vi "RPC Method RouteGuide RecordRoute.vi"(3 "error in (no error)":errorcluster, 4 "gRPCid in":T2, 5 "DNL_LabVIEW Object in":refnum<class "RouteGuideImpl.lvclass">) -> (0 "error out":errorcluster, 1 "gRPCid out":T2, 2 "DNL_LabVIEW Object out":refnum<class "RouteGuideImpl.lvclass">)   [LabVIEW 2019, in "UserCode_impl_server.lvlib" / "RouteGuideImpl.lvclass"]
uses:
  RouteGuideImpl.lvclass
  <vilib>/gRPC/LabVIEW gRPC Library/Shared/grpcId.ctl
  Generated_stub_server/RPC Messages/routeguide_RouteSummary.ctl
  Generated_stub_server/RPC Messages/routeguide_Point.ctl
  Generated_stub_server/Generated_stub_server.lvlib
  Generated_stub_server/RPC Service/RouteGuideStub/RouteGuideStub.lvclass
  <vilib>/gRPC/LabVIEW gRPC Library/grpc-lvsupport-release.lvlib
panel:
  in  "?":T1
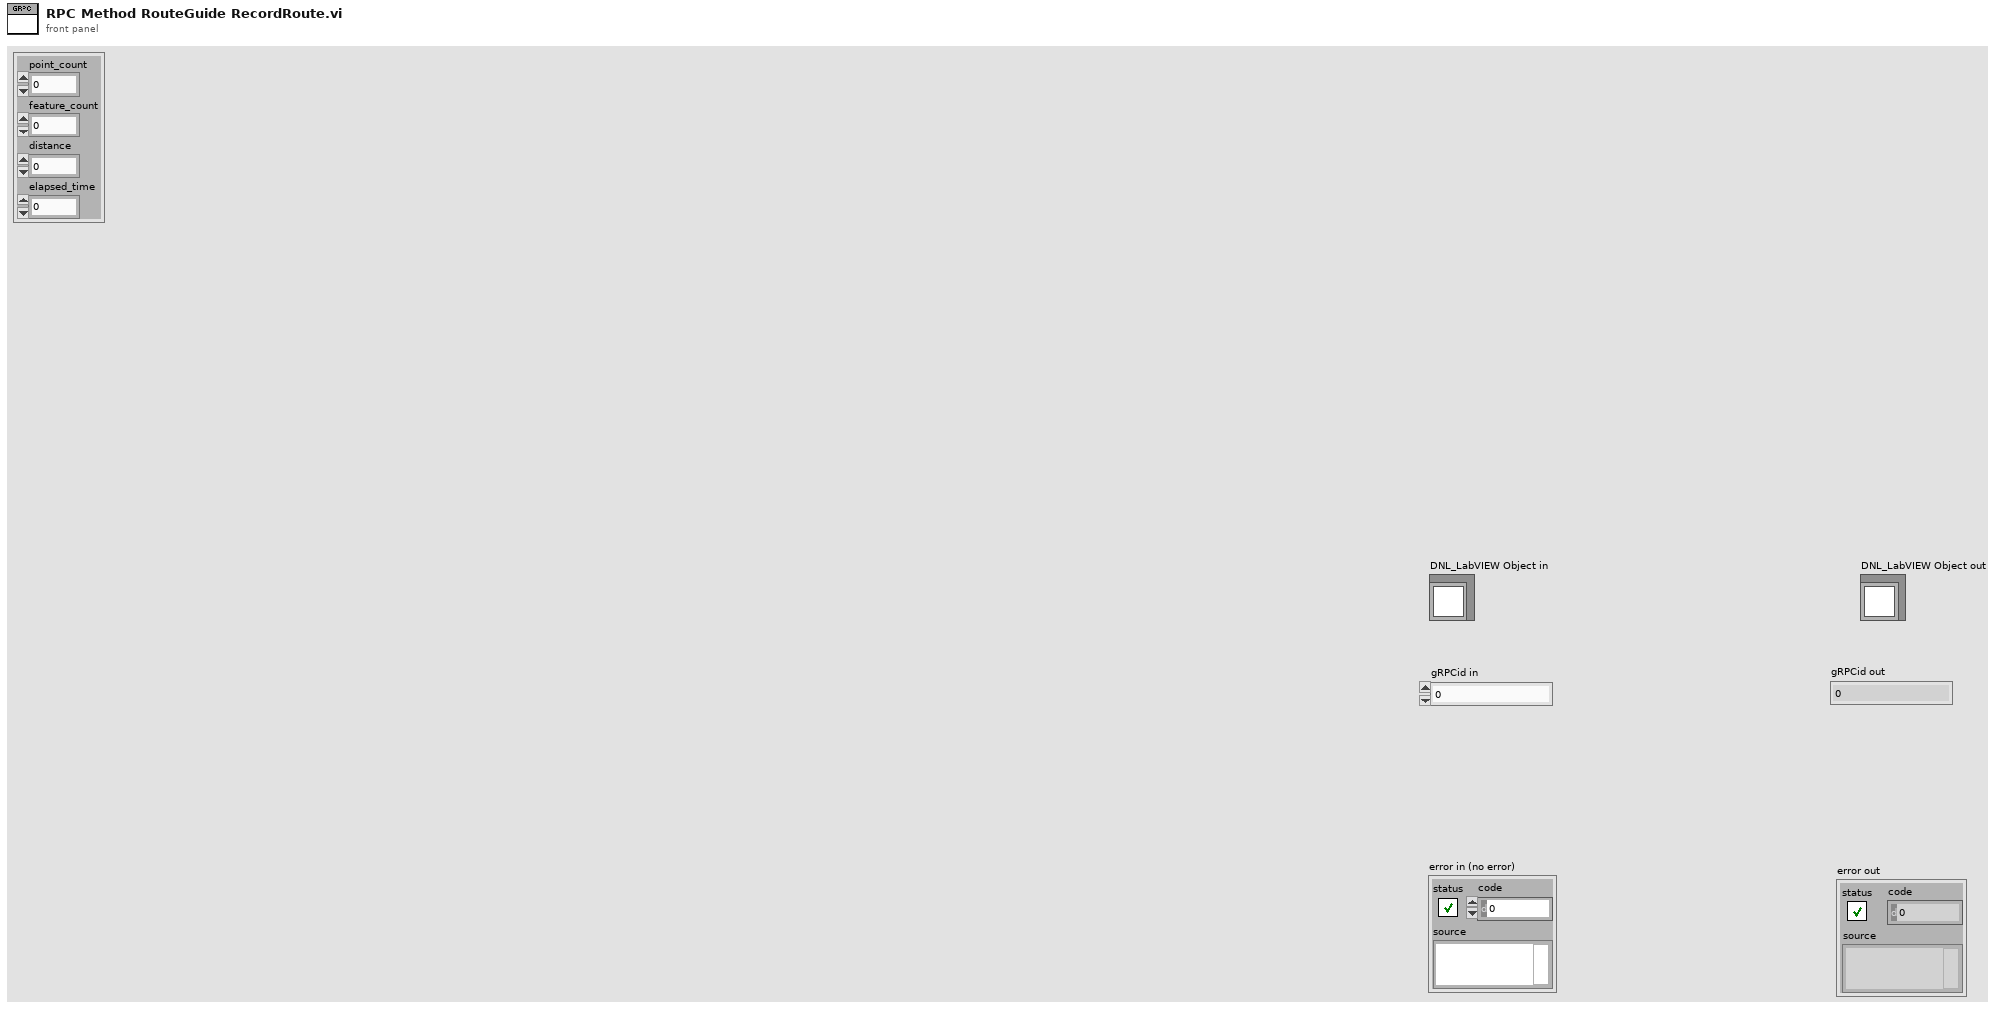
[diagram p1: front panel]
types:
  T1 = typedef "Generated_stub_server.lvlib/routeguide_RouteSummary.ctl" = cluster{"point_count":i32, "feature_count":i32, "distance":i32, "elapsed_time":i32}
  T2 = typedef "grpc-lvsupport-release.lvlib/grpcId.ctl" = u64
  T3 = typedef "Generated_stub_server.lvlib/routeguide_Point.ctl" = cluster{"latitude":i32, "longitude":i32}
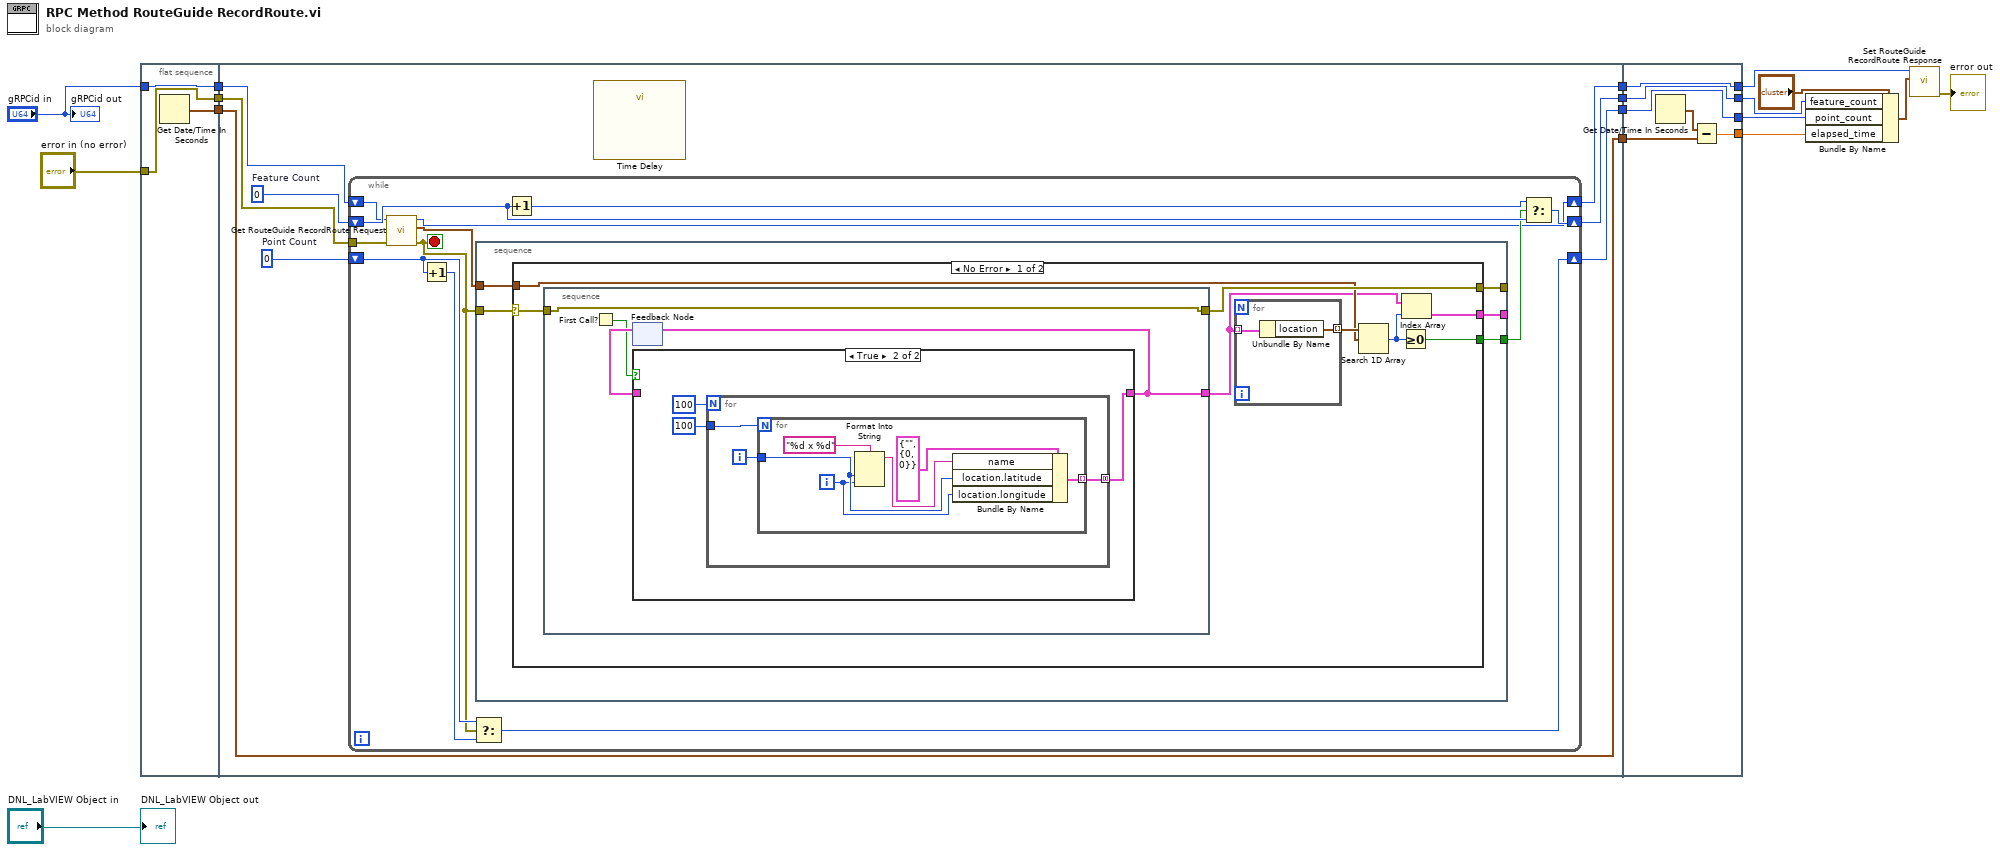
[diagram p0: block diagram]
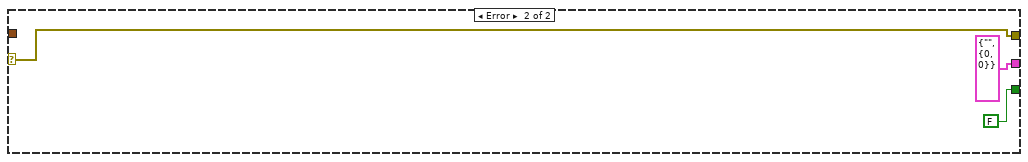
[diagram p3: hidden frame]
diagram:
  n1 = flat-sequence {
    tunnel: [w20] -> w16
    tunnel: "gRPCid in" -> [w19]
    tunnel: [w19] -> w4
    tunnel: "error in (no error)" -> [w18]
    tunnel: [w18] -> w2
    tunnel: [w28] -> w15
    tunnel: [w24] -> w14
    tunnel: [w26] -> w13
    tunnel: w16 -> [w23]
    tunnel: [w23] -> w12
    tunnel: w4 -> [w22]
    tunnel: w2 -> [w21]
    tunnel: [w80] -> w11
    tunnel: [w81] -> w6
    tunnel: w15 -> [w81]
    tunnel: w14 -> [w80]
    tunnel: [w79] -> w10
    tunnel: w13 -> [w79]
    tunnel: w12 -> [w77]
    tunnel: [w76] -> w9
    frame #0 {
      n2 = Get Date/Time In Seconds() -> (seconds since 1Jan1904=w20:timestamp)
    }
    frame #1 {
      w25 = 0  # Point Count
      w27 = 0  # Feature Count
      n3 = while {
        shift-right: [w32] -> w28
        shift-left: w22 -> [w33]
        shift-right: [w40] -> w26
        shift-left: w27 -> [w39]
        shift-right: [w36] -> w24
        shift-left: w25 -> [w34]
        tunnel: w21 -> [w29]
        stop <- w31 stop-if-true
        n4 = call "Get RouteGuide RecordRoute Request.vi"("error in (no error)"=w29, "gRPCid"=w33) -> ("error out"=w31:errorcluster, "Message Data"=w30:T3, "gRPCid out"=w32:T2)  [unwired: 7 in]
        n5 = Increment(x=w34) -> (x+1=w35:i32)
        n6 = Select(t=w34, s=w31, f=w35) -> (s? t:f=w36:i32)
        n7 = stacked-sequence {
          tunnel: [w42] -> _
          tunnel: [w45] -> w37
          tunnel: [w44] -> _
          tunnel: w31 -> [w41]
          tunnel: w30 -> [w43]
          frame #0 {
            n8 = case shown="No Error" w41 {
              selector: w41 -> [w53 w75]
              tunnel: [w52 w75] -> w42
              tunnel: w43 -> [w50 _]
              tunnel: [w47 cluster{"name":string, "routeguide_Point":T3} {"name"="", "routeguide_Point"={"latitude"=0, "longitude"=0}} ("routeguide_Feature")] -> w44
              tunnel: [w46 FALSE] -> w45
              frame No Error {
                n9 = stacked-sequence {
                  tunnel: [w54] -> w52
                  tunnel: [w56] -> w49
                  tunnel: w53 -> [w54]
                  frame #0 {
                    n10 = First Call?() -> (First Call?: T/F=w55:bool)
                    n11 = feedback #1() -> (w57:cluster{"name":string, "location":T3}[])  [unwired: 1 in]
                    n12 = case shown="True" w55 {
                      tunnel: [w58 w60] -> w56
                      tunnel: w57 -> [w58 _]
                      frame False {
                      }
                      frame True {
                        n13 = for {
                          N: 100 -> [_]
                          tunnel: [w63] -> w60 mode=concatenating
                          tunnel: 100 -> [w62]
                          i -> [w64]
                          n14 = for {
                            N: w62 -> [_]
                            tunnel: w64 -> [w67]
                            tunnel: [w65] -> w63 mode=indexing
                            i -> [w66]
                            n15 = Format Into String(format string="%d x %d", w67, w66) -> (resulting string=w68:string)  [unwired: 2 in, 1 out]
                            n16 = Bundle By Name(cluster=cluster{"name":string, "location":T3} {"name"="", "location"={"latitude"=0, "longitude"=0}} ("routeguide_Feature"), "name"=w68, "location.latitude"=w67, "location.longitude"=w66) -> (w65:cluster{"name":string, "location":T3})
                          }
                        }
                      }
                    }
                    n17 = feedback-in #1(w56) -> ()
                  }
                }
                n18 = for {
                  tunnel: w49 -> [w72] mode=indexing
                  tunnel: [w71] -> w51 mode=indexing
                  n19 = Unbundle By Name(w72) -> ("location"=w71:T3)
                }
                n20 = Search 1D Array(1D array=w51, element=w50) -> (index of element=w48:i32)  [unwired: 1 in]
                n21 = Greater Or Equal To 0?(x=w48) -> (x >= 0?=w46:bool)
                n22 = Index Array(array=w49, index=w48) -> (element=w47:cluster{"name":string, "location":T3})
              }
              frame Error {
              }
            }
          }
        }
        n23 = Increment(x=w39) -> (x+1=w38:i32)
        n24 = Select(t=w38, s=w37, f=w39) -> (s? t:f=w40:i32)
      }
      n25 = call "Time Delay"() -> ()  [unwired: 11 in, 1 out]
    }
    frame #2 {
      n26 = Get Date/Time In Seconds() -> (seconds since 1Jan1904=w78:timestamp)
      n27 = Subtract(x=w78, y=w77) -> (x-y=w76:dbl)
    }
  }
  n28 = Bundle By Name(cluster="?", "feature_count"=w10, "point_count"=w11, "elapsed_time"=w9) -> (w7:T1)
  n29 = call "Set RouteGuide RecordRoute Response.vi"("Message Data"=w7, "gRPCid in"=w6) -> ("error out"=→"error out":errorcluster)  [unwired: 9 in]
  "DNL_LabVIEW Object out" <- "DNL_LabVIEW Object in"
  "gRPCid out" <- "gRPCid in"
